vi "TextControlledInstrumControlToCommandMultiSub.vi"(8 "Offset in (0)":i32, 9 "Command Array":string[](array[string]), 10 "Control Array":refnum<vi>[](array[refnum]), 11 "ControlToCommand in":map{refnum<vi>, string[]}(c390)) -> (0 "Offset out":i32, 3 "ControlToCommand out":map{refnum<vi>, string[]}(c390))   [LabVIEW 2020]
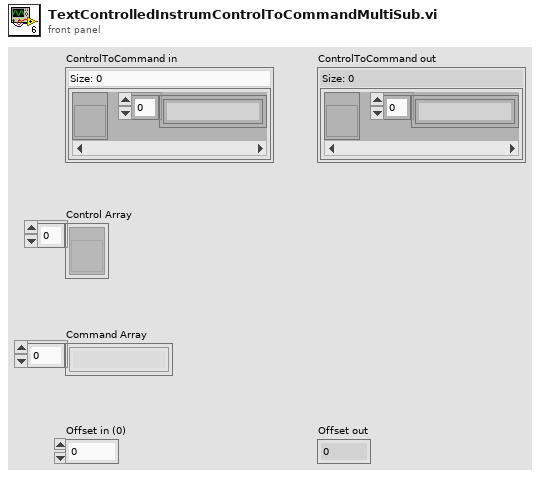
[diagram p1: front panel]
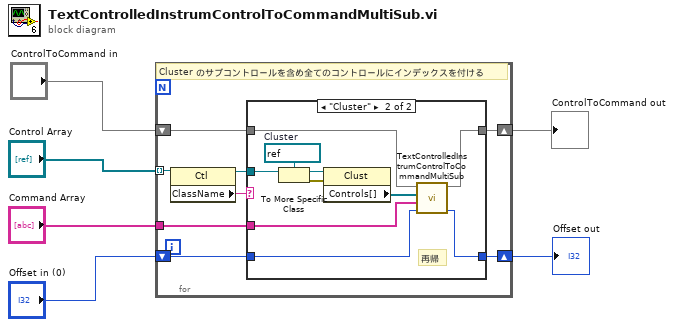
[diagram p0: block diagram]
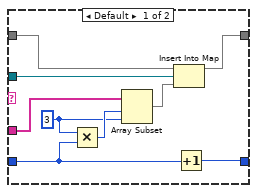
[diagram p2: hidden frame]
diagram:
  n1 = for {
    tunnel: "Control Array" -> [w14] mode=indexing
    shift-right: [w10] -> w5
    shift-left: "Offset in (0)" -> [w11]
    shift-right: [w8] -> w6
    shift-left: "ControlToCommand in" -> [w9]
    tunnel: "Command Array" -> [w7]
    # "Cluster のサブコントロールを含め全てのコントロールにインデックスを付ける"
    n2 = property class="Ctl"(reference=w14) -> (reference out=w12:refnum<vi>, "ClassName"=w13:string)  [unwired: 1 in, 1 out]
    n3 = case shown="\"Cluster\"" w13 {
      tunnel: w12 -> [w20 w33]
      tunnel: w11 -> [w19 w26]
      tunnel: [w23 w25] -> w10
      tunnel: w9 -> [w22 w28]
      tunnel: [w21 w27] -> w8
      tunnel: w7 -> [w17 w24]
      frame Default {
        w15 = 3
        n4 = Multiply(x=w15, y=w19) -> (x*y=w16:i32)
        n5 = Array Subset(array=w17, index=w16, length=w15) -> (w18:string[])
        n6 = Insert Into Map(map in=w22, key=w20, value=w18) -> (map out=w21:map{refnum<vi>, string[]})  [unwired: 2 out]
        n7 = Increment(x=w19) -> (x+1=w23:i32)
      }
      frame "Cluster" {
        w30 = refnum<vi> refnum  # Cluster
        # "再帰"
        n8 = To More Specific Class(target class=w30, reference=w33) -> (specific class reference=w32:refnum<vi>, error out=w31:errorcluster)  [unwired: 1 in]
        n9 = property class="Clust"(reference=w32, error in=w31) -> ("Controls[]"=w29:refnum<vi>[])  [unwired: 2 out]
        n10 = call "TextControlledInstrumControlToCommandMultiSub.vi"("Offset in (0)"=w26, "Command Array"=w24, "Control Array"=w29, "ControlToCommand in"=w28) -> ("Offset out"=w25:i32, "ControlToCommand out"=w27:map{refnum<vi>, string[]})  [unwired: 6 in]
      }
    }
  }
  "Offset out" <- w5
  "ControlToCommand out" <- w6
